vi "sonar analog distance.vi"(7 "AIDeviceRef in":T1, 9 "Average Bits":u8=3 max=15, 10 "Samples Per Second":dbl=1000.0, 11 "Scaling factor (V/in)":dbl=0.0098) -> (0 "error out":errorcluster, 2 "AIDeviceRef out":T1, 3 "distance":dbl(slide)=125.0 scale=0.0..250.0 scale format="%3d")   [LabVIEW 2011]
uses:
  <vilib>/Rock Robotics/WPI/AnalogChannel/WPI_AnalogChannelDevRef.ctl
  <vilib>/Rock Robotics/SystemInterfaces/Typedef/FPGA_TypedefAnalogModule.ctl
  <vilib>/Rock Robotics/SystemInterfaces/AI/FPGA_AIChannel.ctl
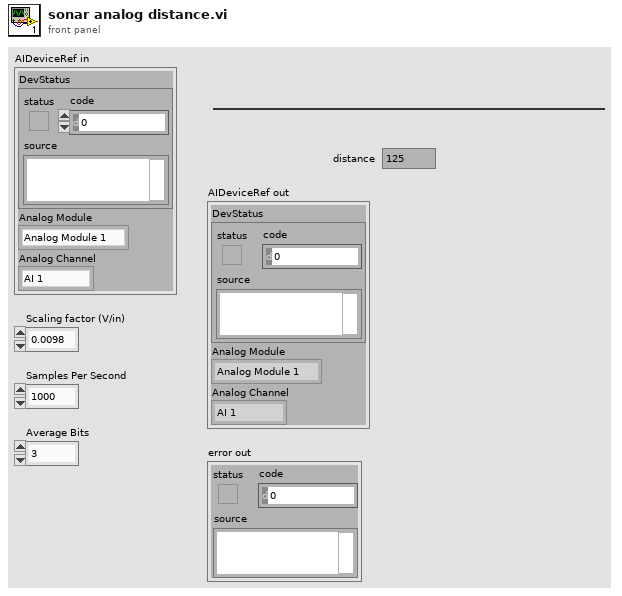
[diagram p1: front panel]
types:
  T1 = typedef "WPI_AnalogChannelDevRef.ctl" = cluster{"DevStatus":errorcluster, "Analog Module":T2, "Analog Channel":T3}
  T2 = typedef "FPGA_TypedefAnalogModule.ctl" = enum16{"Analog Module 1", "Analog Module 2"}
  T3 = typedef "FPGA_AIChannel.ctl" = enum8{"AI 1", "AI 2", "AI 3", "AI 4", "AI 5", "AI 6", "AI 7", "AI 8", "Invalid"}
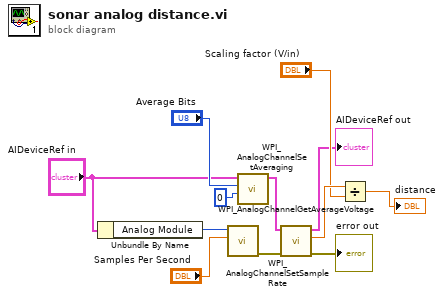
[diagram p0: block diagram]
diagram:
  n1 = Unbundle By Name("AIDeviceRef in") -> ("Analog Module"=w1:T2)
  n2 = call <vilib>:"WPI_AnalogChannelSetSampleRate.vi"("Samples Per Second"="Samples Per Second", "Analog Module (Module 1)"=w1) -> ("error out"=w12:errorcluster)  [unwired: 2 in, 7 out]
  n3 = call <vilib>:"WPI_AnalogChannelSetAveraging.vi"("OversampleBits"=u8 0, "AverageBits"="Average Bits", "AIDeviceRef"="AIDeviceRef in") -> ("AIDeviceRef"=w11:T1)  [unwired: 1 in, 7 out]
  n4 = call <vilib>:"WPI_AnalogChannelGetAverageVoltage.vi"("error in (no error)"=w12, "AIDeviceRef"=w11) -> ("error out"=→"error out":errorcluster, "Voltage"=w9:dbl, "AIDeviceRef"=→"AIDeviceRef out":T1)  [unwired: 7 out]
  n5 = Divide(x=w9, y="Scaling factor (V/in)") -> (x/y=→"distance":dbl)
